vi "SecurityNode.vi"() -> ()   [LabVIEW 2011]
doc: "Host interface for JeeNode based Security Node\n\nInstructions: Attach a JeeNode programmed with the RF12demo example via a USB adapter. Set the COM port in \"VISA resource name\" and run.\n\nLicense: http://opensource.org/licenses/mit-license.php\n\nCopyright (c) 2012 Ken Sharp"
uses:
  <vilib>/Instr/_visa.llb/VISA Configure Serial Port (Instr).vi
panel:
  in  "Sensor Update":bool
  in  "Siren":bool
  out "System Armed":bool
  out "Emergency?":bool
  out "Alarm?":bool
  in  "Arm System":bool
  in  "Arm motion sensor":bool
  out "panic button":bool
  out "motion sensor":bool
  out "front door":bool
  out "back door":bool
  out "garage door":bool
  out "Thermometer":dbl(slide) scale=0.0..100.0 scale format="%#_3g"
  in  "stop":bool
  in  "VISA resource name":refnum<visa-resource-name>
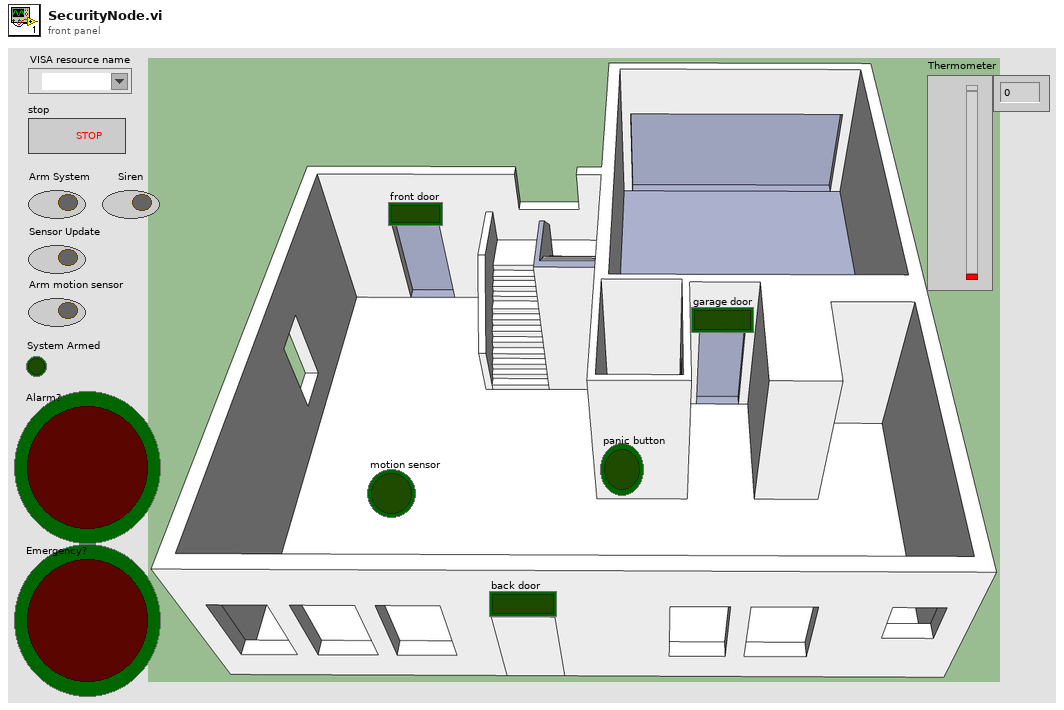
[diagram p1: front panel]
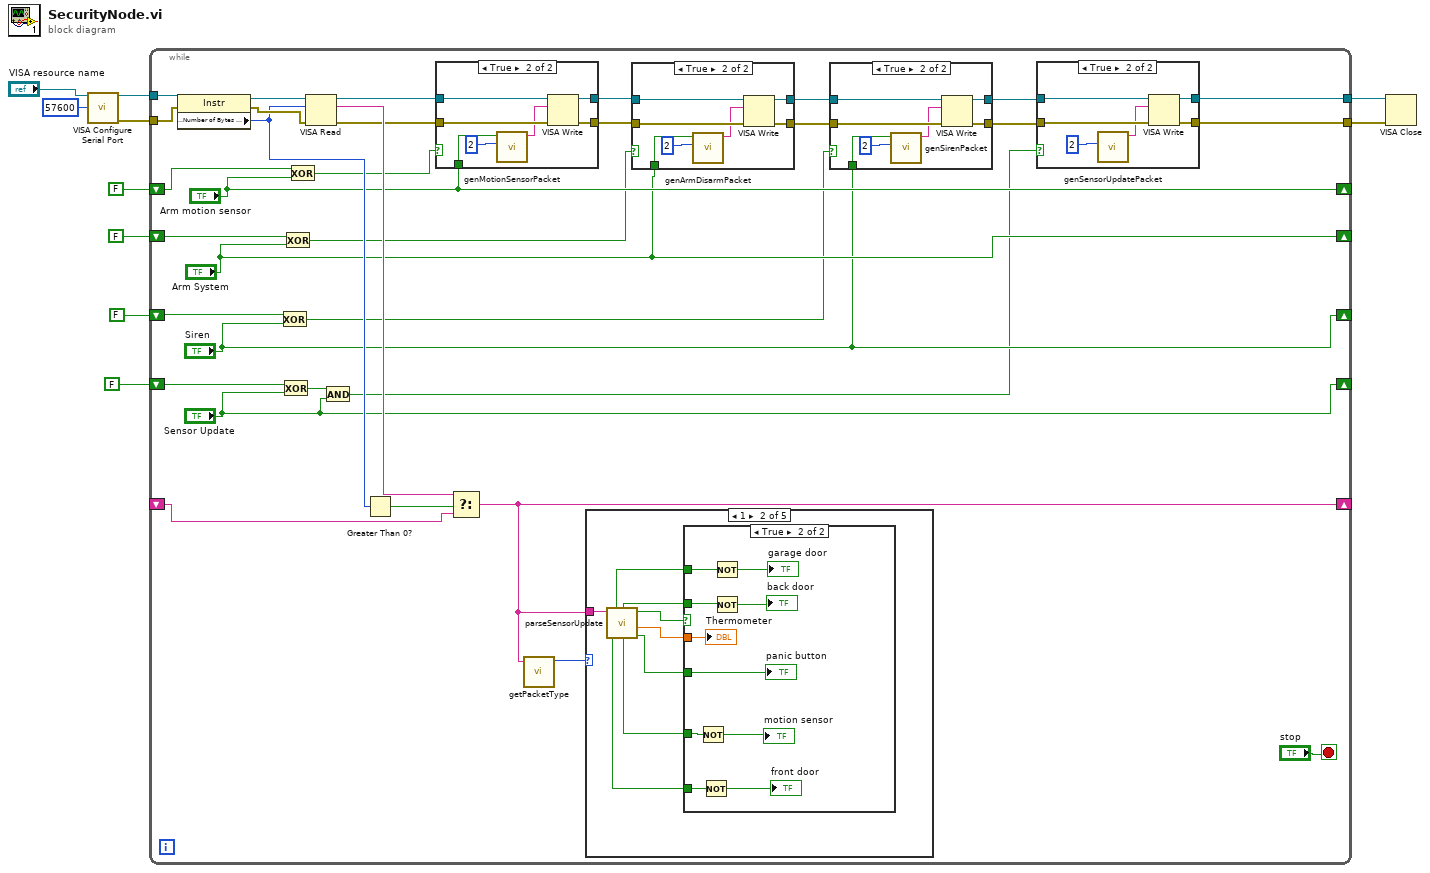
[diagram p0: block diagram]
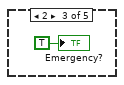
[diagram p7: hidden frame]
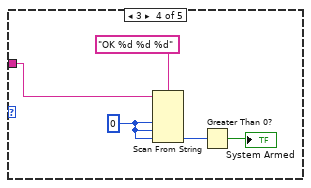
[diagram p8: hidden frame]
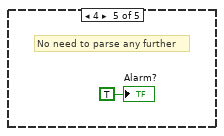
[diagram p9: hidden frame]
diagram:
  n1 = call-poly "VISA Configure Serial Port"("VISA resource name"="VISA resource name", "baud rate (9600)"=u32 57600) -> ("VISA resource name out"=w9:refnum<visa-resource-name>, "error out"=w8:errorcluster)  [unwired: 12 in]
  n2 = while {
    tunnel: w9 -> [w44]
    tunnel: w8 -> [w42]
    shift-right: [w30] -> _
    shift-left: _ -> [w36]
    shift-right: ["Arm motion sensor"] -> _
    shift-left: FALSE -> [w32]
    shift-right: ["Arm System"] -> _
    shift-left: FALSE -> [w26]
    shift-right: ["Siren"] -> _
    shift-left: FALSE -> [w22]
    shift-right: ["Sensor Update"] -> _
    shift-left: FALSE -> [w23]
    tunnel: [w16] -> w2
    tunnel: [w15] -> w1
    stop <- "stop" stop-if-true
    n3 = property class="Instr"(reference=w44, error in=w42) -> (reference out=w43:refnum<visa-resource-name>, error out=w40:errorcluster, "Serial Settings:Number of Bytes at Serial Port"=w38:u32)
    n4 = Exclusive Or(1:"Siren", 2:w22) -> (0:w21:bool)
    n5 = Exclusive Or(1:"Sensor Update", 2:w23) -> (0:w13:bool)
    n6 = Exclusive Or(1:"Arm System", 2:w26) -> (0:w25:bool)
    n7 = Exclusive Or(1:"Arm motion sensor", 2:w32) -> (0:w33:bool)
    n8 = VISA Read(VISA resource name=w43, byte count=w38, error in (no error)=w40) -> (VISA resource name out=w34:refnum<visa-resource-name>, read buffer=w39:string, error out=w35:errorcluster)  [unwired: 1 out]
    n9 = And(x=w13, y="Sensor Update") -> (x .and. y?=w11:bool)
    n10 = Greater Than 0?(x=w38) -> (x > 0?=w37:bool)
    n11 = case shown="True" w33 {
      tunnel: w35 -> [w97 w101]
      tunnel: w34 -> [w96 w102]
      tunnel: [w97 w104] -> w27
      tunnel: [w96 w103] -> w28
      tunnel: "Arm motion sensor" -> [_ w99]
      frame False {
      }
      frame True {
        n12 = call "genMotionSensorPacket.vi"("node ID"=u8 2, "state"=w99) -> ("packet string"=w100:string)  [unwired: 9 in]
        n13 = VISA Write(VISA resource name=w102, write buffer=w100, error in (no error)=w101) -> (VISA resource name out=w103:refnum<visa-resource-name>, error out=w104:errorcluster)  [unwired: 1 out]
      }
    }
    n14 = Select(t=w39, s=w37, f=w36) -> (s? t:f=w30:string)
    n15 = call "getPacketType.vi"("read buffer"=w30) -> ("type"=w29:i8)  [unwired: 10 in]
    n16 = case shown="1" w29 {
      tunnel: w30 -> [_ w78 _ w93 _]
      frame -1, Default {
      }
      frame 1 {
        n17 = call "parseSensorUpdate.vi"("read buffer"=w78) -> ("panic button"=w75:bool, "temperature (farenheit)"=w77:dbl, "parse successful?"=w76:bool, "motion sensor"=w74:bool, "back door"=w72:bool, "front door"=w73:bool, "garage door"=w71:bool)  [unwired: 3 in, 1 out]
        n18 = case shown="True" w76 {
          tunnel: w77 -> [_ w88]
          tunnel: w75 -> [_ w82]
          tunnel: w74 -> [_ w80]
          tunnel: w73 -> [_ w86]
          tunnel: w72 -> [_ w85]
          tunnel: w71 -> [_ w87]
          frame False {
          }
          frame True {
            n19 = Not(x=w80) -> (.not. x?=→"motion sensor":bool)
            n20 = Not(x=w86) -> (.not. x?=→"front door":bool)
            n21 = Not(x=w87) -> (.not. x?=→"garage door":bool)
            n22 = Not(x=w85) -> (.not. x?=→"back door":bool)
            "Thermometer" <- w88
            "panic button" <- w82
          }
        }
      }
      frame 2 {
        "Emergency?" <- TRUE ("Emergency?")
      }
      frame 3 {
        w92 = 0 ("default value 1")
        n23 = Scan From String(format string="OK %d %d %d", input string=w93, default 1=w92, default 2=w92, default 3=w92) -> (output 3=w91:i32)  [unwired: 4 in, 3 out]
        n24 = Greater Than 0?(x=w91) -> (x > 0?=→"System Armed":bool)
      }
      frame 4 {
        # "No need to parse any further"
        "Alarm?" <- TRUE ("Alarm?")
      }
    }
    n25 = case shown="True" w25 {
      tunnel: w27 -> [w63 w67]
      tunnel: w28 -> [w62 w68]
      tunnel: [w63 w70] -> w20
      tunnel: [w62 w69] -> w19
      tunnel: "Arm System" -> [_ w65]
      frame False {
      }
      frame True {
        n26 = call "genArmDisarmPacket.vi"("node ID"=u8 2, "state"=w65) -> ("packet string"=w66:string)  [unwired: 9 in]
        n27 = VISA Write(VISA resource name=w68, write buffer=w66, error in (no error)=w67) -> (VISA resource name out=w69:refnum<visa-resource-name>, error out=w70:errorcluster)  [unwired: 1 out]
      }
    }
    n28 = case shown="True" w21 {
      tunnel: w20 -> [w54 w58]
      tunnel: w19 -> [w53 w59]
      tunnel: [w54 w61] -> w17
      tunnel: [w53 w60] -> w18
      tunnel: "Siren" -> [_ w56]
      frame False {
      }
      frame True {
        n29 = call "genSirenPacket.vi"("node ID"=u8 2, "state"=w56) -> ("packet string"=w57:string)  [unwired: 9 in]
        n30 = VISA Write(VISA resource name=w59, write buffer=w57, error in (no error)=w58) -> (VISA resource name out=w60:refnum<visa-resource-name>, error out=w61:errorcluster)  [unwired: 1 out]
      }
    }
    n31 = case shown="True" w11 {
      tunnel: w17 -> [w46 w49]
      tunnel: w18 -> [w45 w50]
      tunnel: [w46 w52] -> w15
      tunnel: [w45 w51] -> w16
      frame False {
      }
      frame True {
        n32 = call "genSensorUpdatePacket.vi"("node ID"=u8 2) -> ("packet string"=w48:string)  [unwired: 10 in]
        n33 = VISA Write(VISA resource name=w50, write buffer=w48, error in (no error)=w49) -> (VISA resource name out=w51:refnum<visa-resource-name>, error out=w52:errorcluster)  [unwired: 1 out]
      }
    }
  }
  n34 = VISA Close(VISA resource name=w2, error in (no error)=w1) -> ()  [unwired: 1 out]
